vi "SR Number Sort.vi"(11 "list in":T1[](array[typedef]) {"Creation Date" format="%<%x>T"; "Last Updated" format="%<%x>T"}) -> (3 "Array":T1[](array[typedef]) {"Creation Date" format="%<%x>T"; "Last Updated" format="%<%x>T"})   [LabVIEW 2018]
uses:
  Type Defs/SR Cluster.ctl
  Type Defs/SR Status.ctl
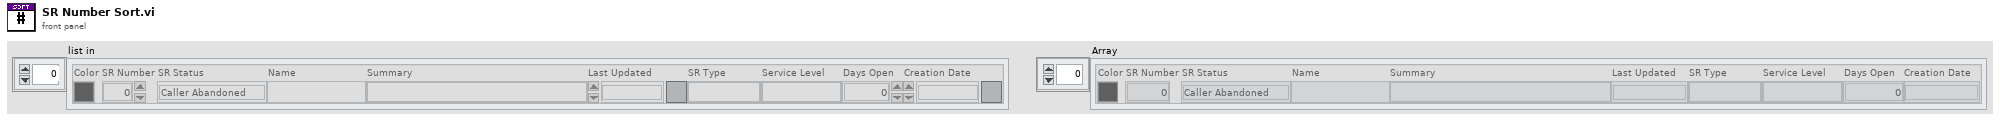
[diagram p1: front panel]
types:
  T1 = typedef "SR Cluster.ctl" = cluster{"Color":u32, "SR Number":i32, "SR Status":T2, "Name":string, "Summary":string, "Last Updated":timestamp, "SR Type":string, "Service Level":string, "Days Open":dbl, "Creation Date":timestamp}
  T2 = typedef "SR Status.ctl" = enum16{"Caller Abandoned", "Created in Error", "Expired", "Forum Resolved AE", "Forum Resolved Customer", "IN WORK", "IN WORK Collab with AES", "IN WORK Collab with PSE", "IN WORK Collab with SE", "IN WORK Customer Added Note", "IN WORK Escalation", "IN WORK Wait on Customer", "Open", "Potentially Resolved", "Presumed Resolved", "RMA Approved for Return", "RMA Closed", "RMA Closed - DOA", "RMA In Progress", "RMA Open", "RMA Waiting on Customer", "Resolved", "Passed Off"}
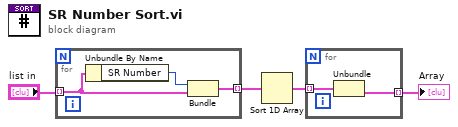
[diagram p0: block diagram]
diagram:
  n1 = for {
    tunnel: "list in" -> [w6] mode=indexing
    tunnel: [w7] -> w1 mode=indexing
    n2 = Unbundle By Name(w6) -> ("SR Number"=w5:i32)
    n3 = Bundle("SR Number"=w5, "SR Cluster"=w6) -> (w7:cluster{"SR Number":i32, "SR Cluster":T1})  [unwired: 1 in]
  }
  n4 = Sort 1D Array(array=w1) -> (sorted array=w2:cluster{"SR Number":i32, "SR Cluster":T1}[])
  n5 = for {
    tunnel: w2 -> [w9] mode=indexing
    tunnel: [w8] -> w4 mode=indexing
    n6 = Unbundle(w9) -> ("SR Cluster"=w8:T1)  [unwired: 1 out]
  }
  "Array" <- w4
